vi "Read Meter Data.vi"(8 "error in (no error)":errorcluster, 11 "VISA resource name":refnum<visa-resource-name>) -> (0 "error out":errorcluster, 2 "Logged Data":dbl[][](array[numeric]), 3 "VISA resource name out":refnum<visa-resource-name>)   [LabVIEW 2013, in "Watts Up Series.lvlib"]
doc: "Reads the data from the internal meter of the Watts Up device. Outputs a 2D array of values, where each row is its own 1D array of the data points for each different measurement type (Watts,Volts,Amps,etc).\n\n<b>Note:</b> This VI may take several minutes to complete."
uses:
  <instrlib>/Watts Up Series/Watts Up Series.lvlib
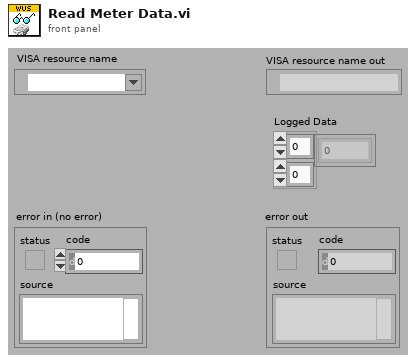
[diagram p1: front panel]
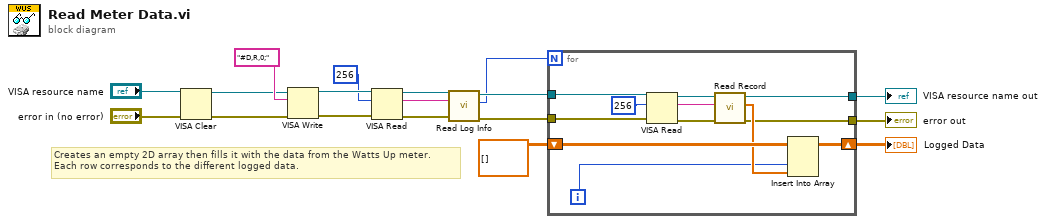
[diagram p0: block diagram]
diagram:
  # "Creates an empty 2D array then fills it with the data from the Watts Up meter.\nEach row corresponds to the different logged data."
  n1 = VISA Clear(VISA resource name="VISA resource name", error in (no error)="error in (no error)") -> (VISA resource name out=w12:refnum<visa-resource-name>, error out=w11:errorcluster)
  n2 = VISA Write(VISA resource name=w12, write buffer="#D,R,0;", error in (no error)=w11) -> (VISA resource name out=w17:refnum<visa-resource-name>, error out=w16:errorcluster)  [unwired: 1 out]
  n3 = VISA Read(VISA resource name=w17, byte count=u32 256, error in (no error)=w16) -> (VISA resource name out=w10:refnum<visa-resource-name>, read buffer=w8:string, error out=w9:errorcluster)  [unwired: 1 out]
  n4 = call <instrlib>:"Read Log Info.vi"("error in (no error)"=w9, "CSV String"=w8, "VISA resource name"=w10) -> ("error out"=w6:errorcluster, "Count"=w4:i32, "VISA resource name out"=w7:refnum<visa-resource-name>)  [unwired: 6 in]
  n5 = for {
    N: w4 -> [_]
    tunnel: w7 -> [w30]
    tunnel: w6 -> [w29]
    tunnel: [w24] -> w5
    shift-right: [w21] -> w2
    shift-left: dbl[][] [] -> [w23]
    tunnel: [w19] -> w1
    i -> [w20]
    n6 = VISA Read(VISA resource name=w30, byte count=u32 256, error in (no error)=w29) -> (VISA resource name out=w27:refnum<visa-resource-name>, read buffer=w26:string, error out=w25:errorcluster)  [unwired: 1 out]
    n7 = call <instrlib>:"Read Record.vi"("error in (no error)"=w25, "CSV String"=w26, "VISA resource name"=w27) -> ("error out"=w19:errorcluster, "Record"=w22:dbl[], "VISA resource name out"=w24:refnum<visa-resource-name>)  [unwired: 6 in]
    n8 = Insert Into Array(array=w23, index (col)=w20, new element=w22) -> (w21:dbl[][])  [unwired: 1 in]
  }
  "VISA resource name out" <- w5
  "error out" <- w1
  "Logged Data" <- w2
